vi "SimpleTest.vi"() -> ()   [LabVIEW 2015]
uses:
  Tek shared libraries/SerialCommunication.lvlib
panel:
  out "Read Buffer":string
  in  "Write Buffer (\"\")":string
  in  "query":bool
  in  "Tab Control":T1(tab)
  in  "output mode":bool
  in  "Output Mode (Arbitrary Waveform)":i32(ring)=1 items=["Arbitrary Waveform"=1, "Arbitrary Sequence"=2]
  in  "output enable":bool
  in  "Channel Name (\"1\")":string="1"
  in  "operation mode":bool
  in  "Operation Mode (Continuous) 2":i32(ring) caption="Operation Mode (Continuous)" items=["Continuous"=0, "Burst"=1, "Gated"=1001, "Sequence"=1002]
  in  "Channel Name (\"1\") 2":string="1"
  in  "set volt":bool
  in  "High Voltage (0.25)":dbl=0.25
  in  "Channel Name (\"1\") 3":string="1" caption="Channel Name (\"1\")"
  in  "Stop Button":bool
  out "error out":errorcluster
  in  "resource name":refnum<k15>
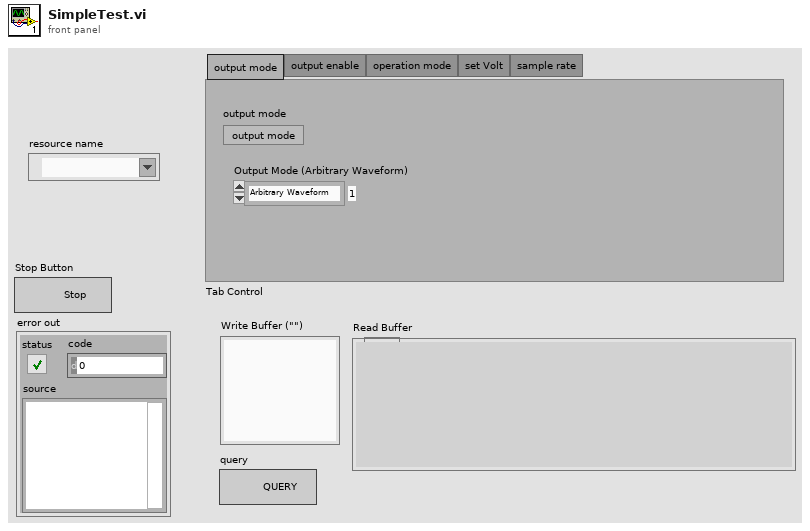
[diagram p1: front panel]
types:
  T1 = enum32{"output mode", "output enable", "operation mode", "set Volt", "sample rate"}
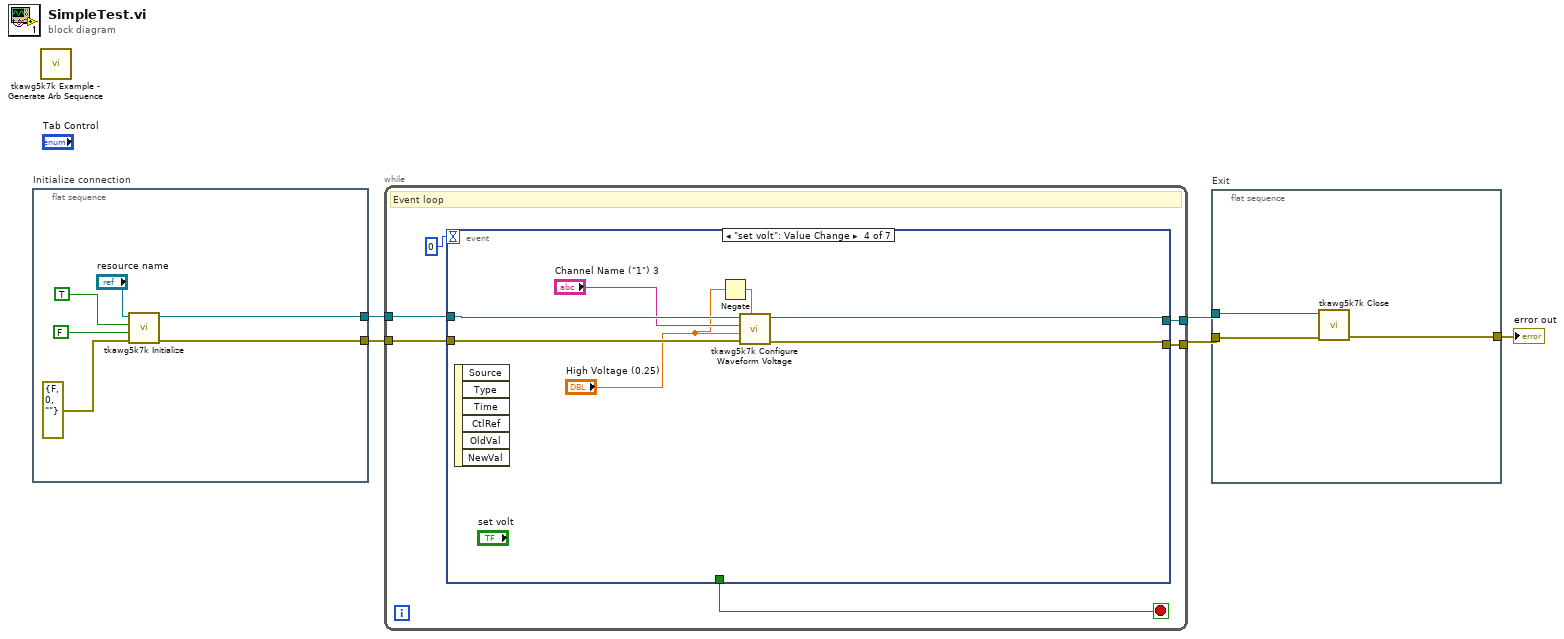
[diagram p0: block diagram]
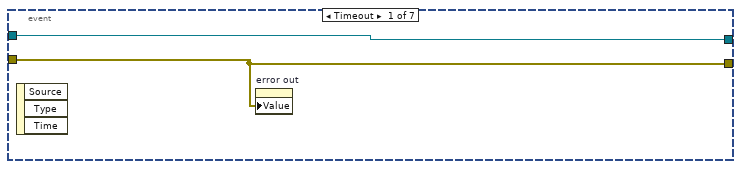
[diagram p2: hidden frame]
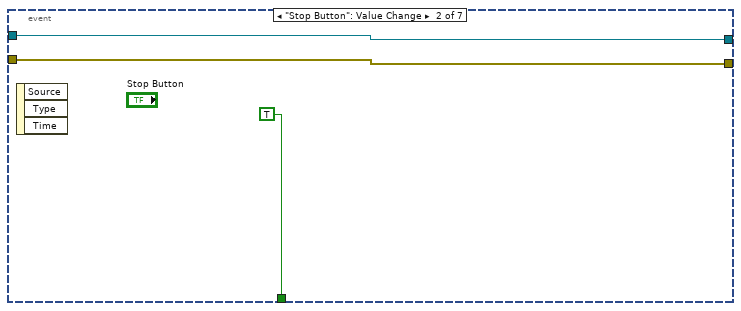
[diagram p3: hidden frame]
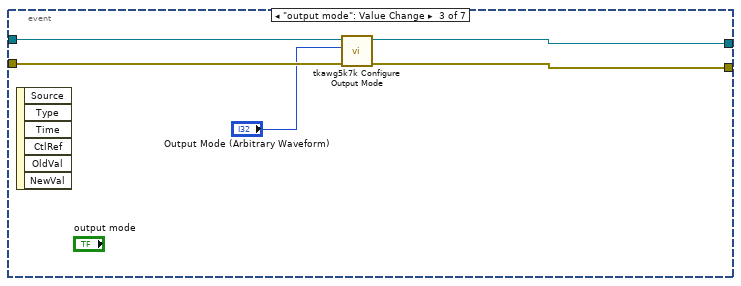
[diagram p4: hidden frame]
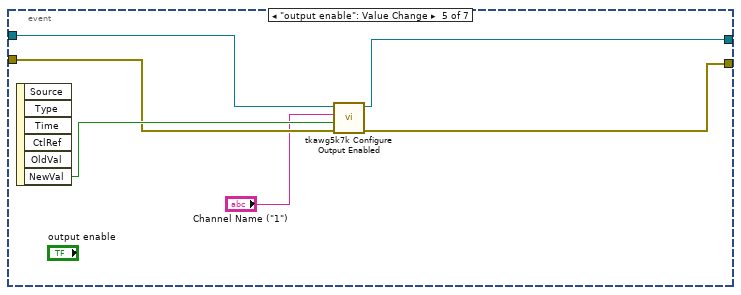
[diagram p5: hidden frame]
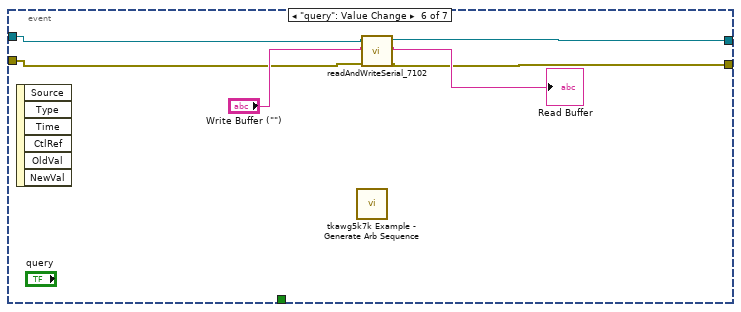
[diagram p6: hidden frame]
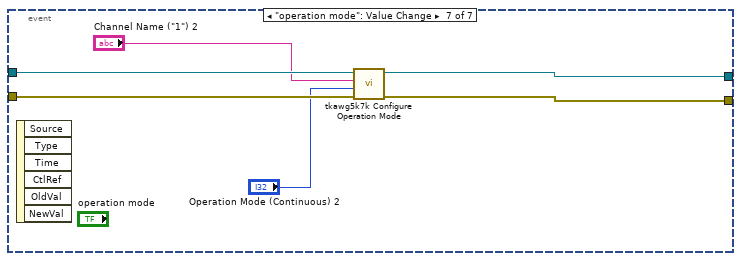
[diagram p7: hidden frame]
diagram:
  n1 = flat-sequence "Initialize connection" {
    tunnel: [w9] -> w5
    tunnel: [w8] -> w4
    frame #0 {
      n2 = call <instrlib>:"tkawg5k7k Initialize.vi"("error in (no error)"=errorcluster {"status"=FALSE, "code"=0, "source"=""}, "Reset Device (Yes)"=FALSE, "ID Query (Yes)"=TRUE, "resource name"="resource name") -> ("error out"=w8:errorcluster, "instrument handle out"=w9:refnum<k15>)  [unwired: 6 in]
    }
  }
  n3 = call <instrlib>:"tkawg5k7k Example - Generate Arb Sequence.vi"() -> ()  [unwired: 12 in]
  n4 = while {
    tunnel: w5 -> [w15]
    tunnel: w4 -> [w13]
    tunnel: [w16] -> w3
    tunnel: [w14] -> w2
    stop <- w12 stop-if-true
    # "Event loop"
    n5 = event shown="[3] \"set volt\": Value Change" {
      selector: _ -> [_ _ _ _ _ _ _]
      dyn-events: _ -> [_ _ _ _ _ _ _]
      timeout: 0 -> [_ _ _ _ _ _ _]
      tunnel: [w19 w21 w24 w33 w37 w43 w51] -> w16
      tunnel: w15 -> [w19 w21 w25 w34 w36 w46 w52]
      tunnel: [w18 w20 w27 w32 w38 w41 w50] -> w14
      tunnel: w13 -> [w18 w20 w26 w31 w39 w44 w49]
      tunnel: [_ TRUE _ _ _ _ _] -> w12
      event Timeout {
        n6 = event-data() -> ()  [unwired: 1 in, 3 out]
        n7 = property on="error out" class="Clust (strict)"("Value"=w18) -> ()  [unwired: 2 in, 2 out]
      }
      event "Stop Button": Value Change {
        n8 = event-data() -> ()  [unwired: 1 in, 3 out]
      }
      event "output mode": Value Change {
        n9 = event-data() -> ()  [unwired: 1 in, 6 out]
        n10 = call <instrlib>:"tkawg5k7k Configure Output Mode.vi"("error in (no error)"=w26, "Output Mode (Arbitrary Waveform)"="Output Mode (Arbitrary Waveform)", "instrument handle"=w25) -> ("error out"=w27:errorcluster, "instrument handle out"=w24:refnum<k15>)  [unwired: 7 in]
      }
      event "set volt": Value Change {
        n11 = event-data() -> ()  [unwired: 1 in, 6 out]
        n12 = Negate(x="High Voltage (0.25)") -> (-x=w28:dbl)
        n13 = call <instrlib>:"tkawg5k7k Configure Waveform Voltage.vi"("Low Voltage (-0.25)"=w28, "error in (no error)"=w31, "High Voltage (0.25)"="High Voltage (0.25)", "Channel Name (\"1\")"="Channel Name (\"1\") 3", "instrument handle"=w34) -> ("error out"=w32:errorcluster, "instrument handle out"=w33:refnum<k15>)  [unwired: 5 in]
      }
      event "output enable": Value Change {
        n14 = event-data() -> ("NewVal"=w40:bool)  [unwired: 1 in, 5 out]
        n15 = call <instrlib>:"tkawg5k7k Configure Output Enabled.vi"("error in (no error)"=w39, "Channel Enabled (True)"=w40, "Channel Name (\"1\")"="Channel Name (\"1\")", "instrument handle"=w36) -> ("error out"=w38:errorcluster, "instrument handle out"=w37:refnum<k15>)  [unwired: 6 in]
      }
      event "query": Value Change {
        n16 = event-data() -> ()  [unwired: 1 in, 6 out]
        n17 = call <instrlib>:"tkawg5k7k Example - Generate Arb Sequence.vi"() -> ()  [unwired: 12 in]
        n18 = call "readAndWriteSerial_7102.vi"("error in (no error)"=w44, "Write Buffer (\"\")"="Write Buffer (\"\")", "instrument handle"=w46) -> ("error out"=w41:errorcluster, "Read Buffer"=→"Read Buffer":string, "instrument handle out"=w43:refnum<k15>)  [unwired: 6 in]
      }
      event "operation mode": Value Change {
        n19 = event-data() -> ()  [unwired: 1 in, 6 out]
        n20 = call <instrlib>:"tkawg5k7k Configure Operation Mode.vi"("error in (no error)"=w49, "Operation Mode (Continuous)"="Operation Mode (Continuous) 2", "Channel Name (\"1\")"="Channel Name (\"1\") 2", "instrument handle"=w52) -> ("error out"=w50:errorcluster, "instrument handle out"=w51:refnum<k15>)  [unwired: 6 in]
      }
    }
  }
  n21 = flat-sequence "Exit" {
    tunnel: w3 -> [w55]
    tunnel: w2 -> [w54]
    tunnel: [w53] -> w1
    frame #0 {
      n22 = call <instrlib>:"tkawg5k7k Close.vi"("error in (no error)"=w54, "instrument handle"=w55) -> ("error out"=w53:errorcluster)  [unwired: 9 in]
    }
  }
  "error out" <- w1
